vi "Client Handshake.vi"(8 "error in (no error)":errorcluster, 10 "Client Handshake":T1, 11 "Messaging Server Module in":refnum<class "Messaging Server Module.lvclass">) -> (0 "error out":errorcluster, 3 "Messaging Server Module out":refnum<class "Messaging Server Module.lvclass">)   [LabVIEW 2020, in "Volatus.lvlib" / "Messaging Server Module.lvclass"]
uses:
  Messaging Server Module.lvclass
  Messaging Server Module.lvclass/Messaging Server Module.ctl
  lv-vecto/Vecto/proto/TcpClientHello/Data.ctl
  lv-vecto/Vecto/proto/TcpClientHello/TcpClientHello.lvlib
  Messaging Client/Client Handshake.ctl
  Messaging Client/Messaging Server Client.lvclass
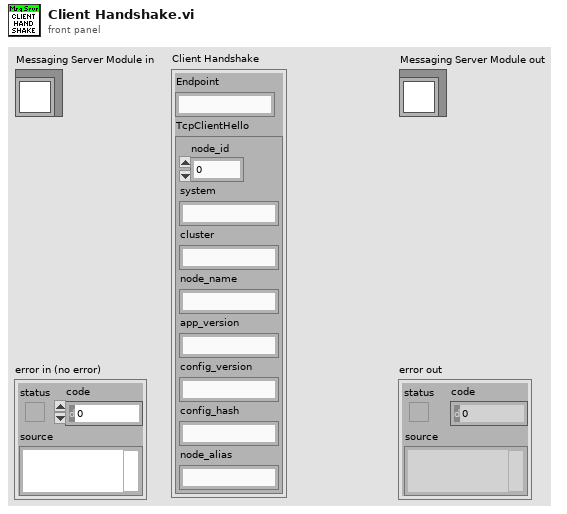
[diagram p1: front panel]
types:
  T1 = typedef "Volatus.lvlib/Messaging Server Client.lvclass/Client Handshake.ctl" = cluster{"Endpoint":string, "TcpClientHello":T2}
  T2 = typedef "TcpClientHello.lvlib/Data.ctl" = cluster{"node_id":u32, "system":string, "cluster":string, "node_name":string, "app_version":string, "config_version":string, "config_hash":string, "node_alias":string}
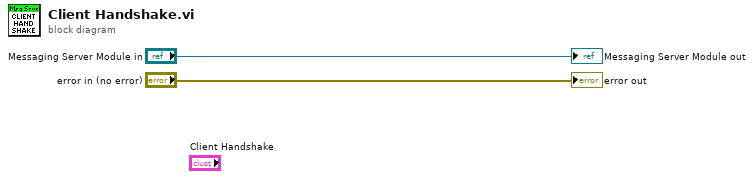
[diagram p0: block diagram]
diagram:
  "error out" <- "error in (no error)"
  "Messaging Server Module out" <- "Messaging Server Module in"
